vi "Apply Heat.vi"(8 "error in (no error)":errorcluster, 10 "Fire (%)":dbl min=0.0 max=100.0 format="%.2f", 11 "Ramp Oven in":refnum<class "Ramp Oven.lvclass">) -> (0 "error out":errorcluster, 3 "Ramp Oven out":refnum<class "Ramp Oven.lvclass">)   [LabVIEW 2021, in "Oven Actor.lvlib" / "Ramp Oven.lvclass"]
uses:
  Ramp Oven.lvclass
  <vilib>/Analysis/NI_AALBase.lvlib
  <vilib>/Analysis/1siggen.llb/Ramp Pattern by Samples.vi
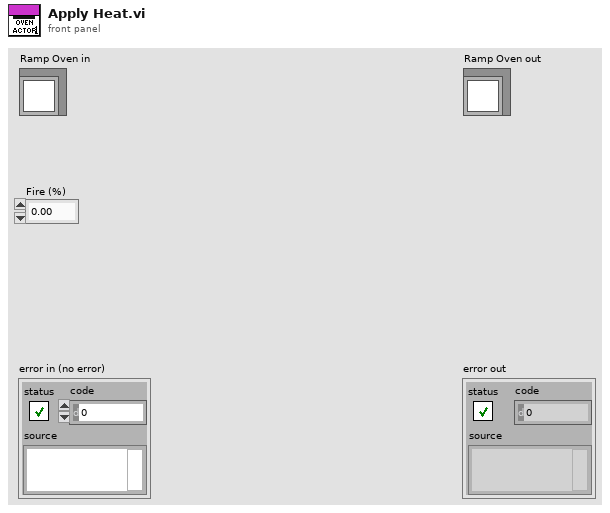
[diagram p1: front panel]
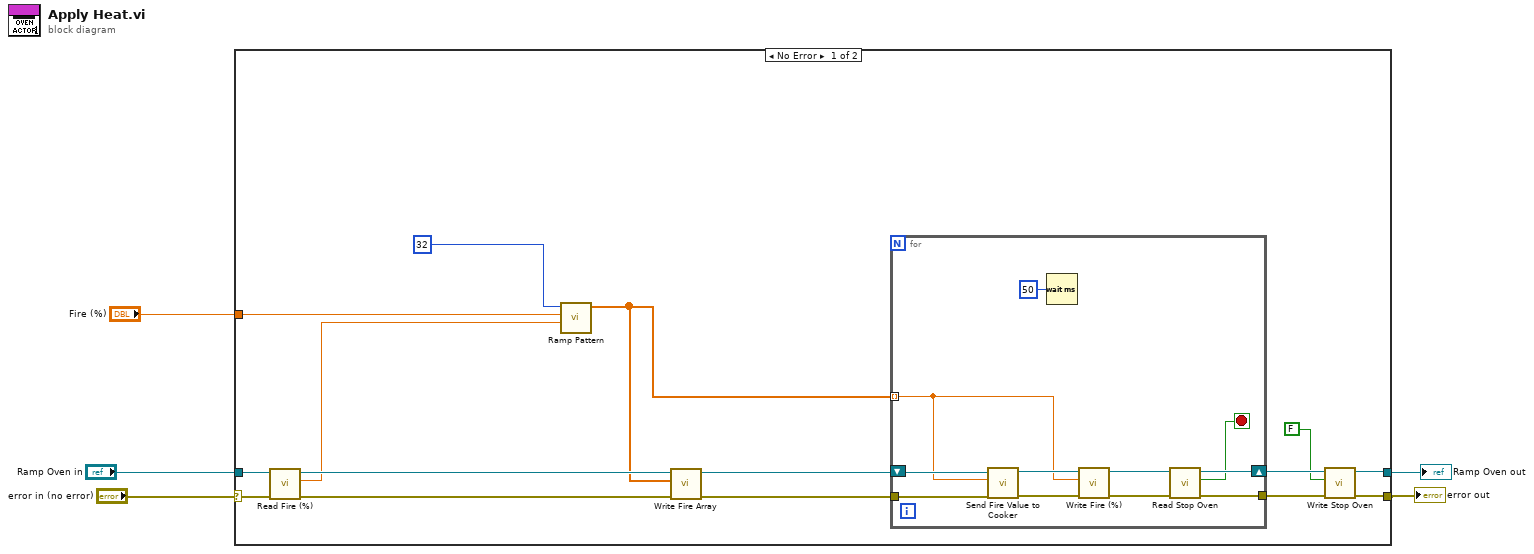
[diagram p0: block diagram]
diagram:
  n1 = case shown="No Error" "error in (no error)" {
    selector: "error in (no error)" -> [w20 w32]
    tunnel: [w12 w32] -> w4
    tunnel: "Ramp Oven in" -> [w18 w33]
    tunnel: [w10 w33] -> w2
    tunnel: "Fire (%)" -> [w8 _]
    frame No Error {
      n2 = call-dynamic "Read Fire (%).vi"("error in (no error)"=w20, "Oven Actor in"=w18) -> ("error out"=w19:errorcluster, "Fire (%)"=w7:dbl, "Oven Actor out"=w17:refnum<class "Ramp Oven.lvclass">)  [unwired: 7 in]
      n3 = call-poly <vilib>:"Ramp Pattern.vi"("start"=w7, "end"=w8, "samples"=32) -> ("Ramp Pattern"=w16:dbl[])  [unwired: 7 in, 1 out]
      n4 = call-dynamic "Write Fire Array.vi"("error in (no error)"=w19, "Fire Array"=w16, "Oven Actor in"=w17) -> ("error out"=w14:errorcluster, "Oven Actor out"=w15:refnum<class "Ramp Oven.lvclass">)  [unwired: 7 in]
      n5 = for {
        tunnel: w16 -> [w21] mode=indexing
        tunnel: w14 -> [w31]
        tunnel: [w27] -> w13
        shift-right: [w26] -> w11
        shift-left: w15 -> [w30]
        stop <- w25 stop-if-true
        n6 = call-dynamic "Send Fire Value to Cooker.vi"("error in (no error)"=w31, "Fire (%)"=w21, "Oven Actor in"=w30) -> ("error out"=w29:errorcluster, "Oven Actor out"=w23:refnum<class "Ramp Oven.lvclass">)  [unwired: 7 in]
        n7 = Wait (ms)(milliseconds to wait=u32 50) -> ()  [unwired: 1 out]
        n8 = call-dynamic "Write Fire (%).vi"("error in (no error)"=w29, "Fire (%)"=w21, "Oven Actor in"=w23) -> ("error out"=w24:errorcluster, "Oven Actor out"=w22:refnum<class "Ramp Oven.lvclass">)  [unwired: 7 in]
        n9 = call-dynamic "Read Stop Oven.vi"("error in (no error)"=w24, "Oven Actor in"=w22) -> ("error out"=w27:errorcluster, "Stop Oven"=w25:bool, "Oven Actor out"=w26:refnum<class "Ramp Oven.lvclass">)  [unwired: 7 in]
      }
      n10 = call-dynamic "Write Stop Oven.vi"("error in (no error)"=w13, "Stop Oven"=FALSE, "Oven Actor in"=w11) -> ("error out"=w12:errorcluster, "Oven Actor out"=w10:refnum<class "Ramp Oven.lvclass">)  [unwired: 7 in]
    }
    frame Error {
    }
  }
  "error out" <- w4
  "Ramp Oven out" <- w2
